vi "T2_Test_Frequency_Calibration_V2.vi"() -> ()   [LabVIEW 2020]
uses:
  <instrlib>/niFgen/niFgen.llb/niFgen Output Mode.ctl
  <instrlib>/niFgen/niFgen.llb/niFgen Waveform Type.ctl
  <instrlib>/niFgen/niFgen.llb/niFgen_ctl Trigger DigEdge - Edge Values (Ring).ctl
  <instrlib>/niFgen/niFgen.llb/niFgen_ctl Trigger Source Values (Ring).ctl
  <instrlib>/niFgen/niFgen.llb/niFgen Trigger Mode.ctl
  <instrlib>/niScope/Controls/niScope acquisition type.ctl
  <instrlib>/niScope/Controls/niScope trigger slope.ctl
  <instrlib>/niScope/Controls/niScope trigger source.ctl
  <vilib>/Utility/file.llb/Read Delimited Spreadsheet (DBL).vi
  <instrlib>/niFgen/niFgen.llb/niFgen Create Waveform (DBL).vi
  <instrlib>/niScope/Configure/Trigger/niScope Configure Trigger Edge.vi
  <instrlib>/niFgen/niFgen.llb/niFgen Configure Digital Edge Start Trigger.vi
  <instrlib>/niScope/Acquire/Fetch/niScope Fetch Cluster.vi
panel:
  out "Pulse Echos - Current Scan":waveform(dbl)(graph)={"t0"=timestamp(0 s since 1904-01-01), "dt"=0.0025142857142857146, "Y"=array[865 elements]} caption="Waveform Graph"
  out "Frequency List (MHz)":dbl[](array[numeric])
  out "Peaks":dbl[](array[numeric])
  in  "Pulse Train File":path=path "D:/Pulse Train - 4s Duration, 3170 Pulses, 1.25ms Tau.txt"
  in  "Starting Frequency":dbl=27440000.0 caption="Frequency" format="%.4p"
  out "Scan Number":i32=1
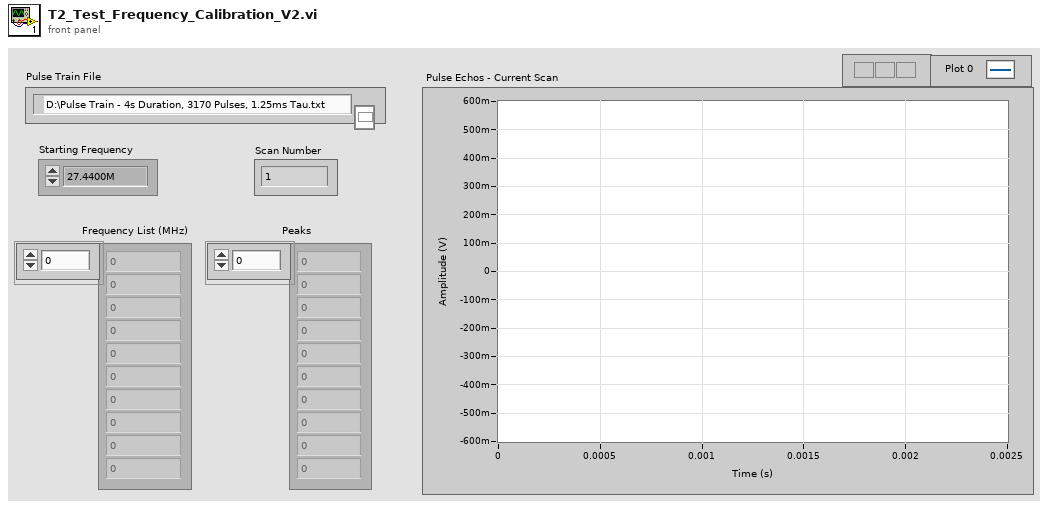
[diagram p1: front panel]
types:
  T1 = typedef "niFgen Output Mode.ctl" = u32
  T2 = typedef "niScope trigger source.ctl" = string
  T3 = typedef "niFgen_ctl Trigger Source Values (Ring).ctl" = string
  T4 = typedef "niScope trigger slope.ctl" = i32
  T5 = typedef "niScope acquisition type.ctl" = i32
  T6 = typedef "niFgen Trigger Mode.ctl" = i32
  T7 = typedef "niFgen_ctl Trigger DigEdge - Edge Values (Ring).ctl" = i32
  T8 = typedef "niFgen Waveform Type.ctl" = i32
  T9 = cluster{"relativeInitialX":dbl, "xIncrement":dbl, "wfm":dbl[]}
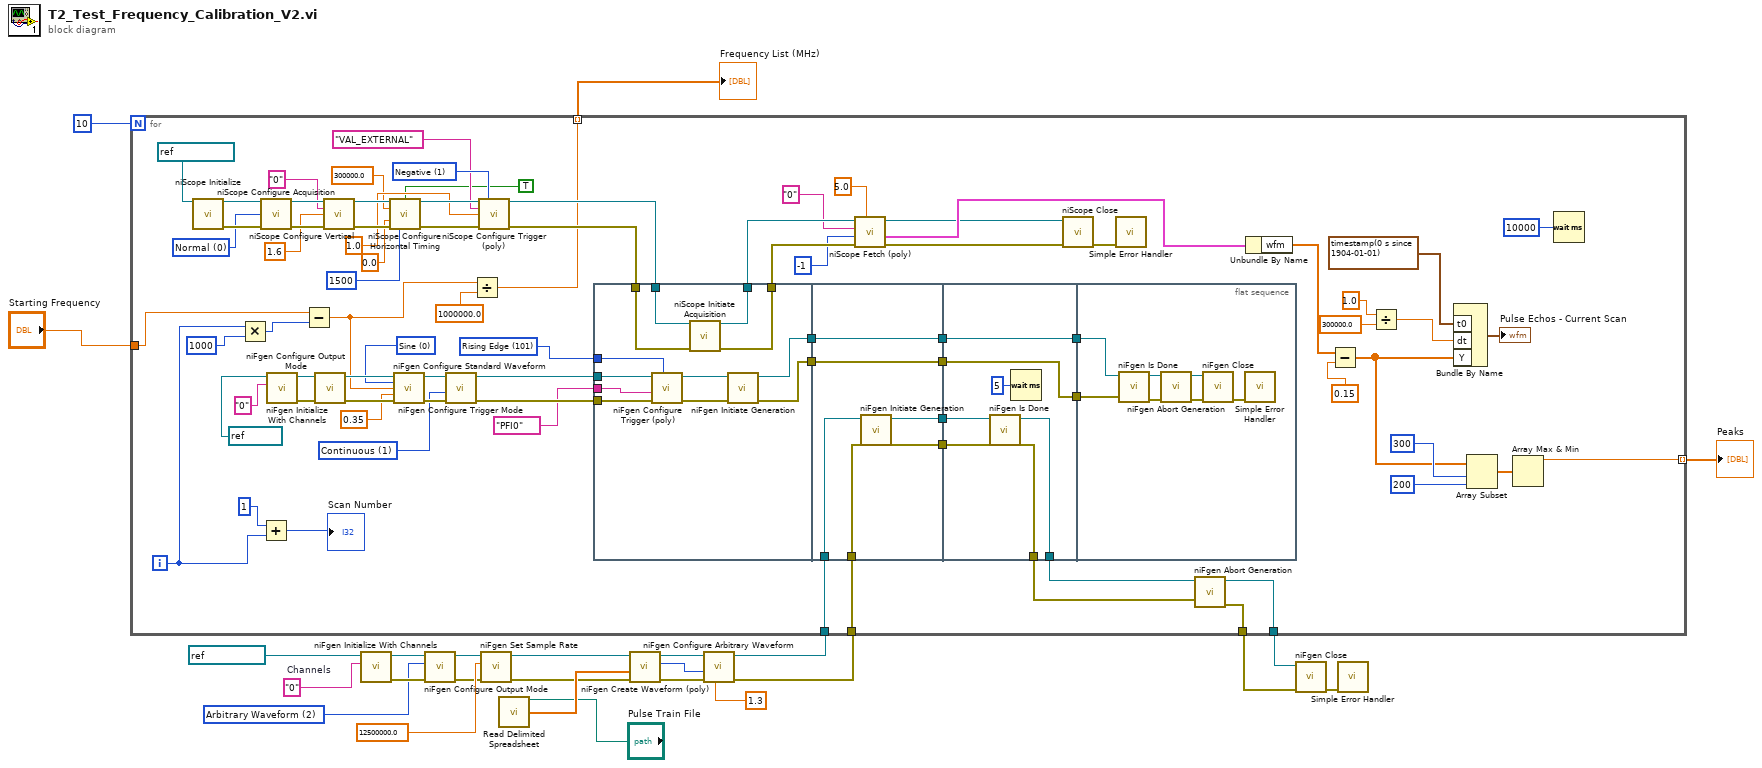
[diagram p0: block diagram]
diagram:
  w11 = "0"  # Channels
  w10 = T1 2 items=["Standard Function", "Frequency List", "Arbitrary Waveform", "Arbitrary Sequence", "Script"] ("output mode")
  n1 = call <instrlib>:"niFgen Initialize With Channels.vi"("Channel Name"=w11, "Resource Name"=refnum<k15> "PXI1Slot3" ("FGEN Resource Name 2")) -> ("error out"=w14:errorcluster, "Instrument Handle Out"=w15:refnum<k15>)  [unwired: 8 in]
  n2 = call <instrlib>:"niFgen Configure Output Mode.vi"("error in (no error)"=w14, "Output Mode (default: 0=Standard Function)"=w10, "Instrument Handle"=w15) -> ("error out"=w18:errorcluster, "Instrument Handle Out"=w17:refnum<k15>)  [unwired: 6 in]
  n3 = call <instrlib>:"niFgen Set Sample Rate.vi"("error in (no error)"=w18, "Sample Rate (Samp/s)"=12500000.0 ("Sample Rate"), "Instrument Handle"=w17) -> ("error out"=w21:errorcluster, "Instrument Handle Out"=w20:refnum<k15>)  [unwired: 7 in]
  n4 = call-poly <vilib>:"Read Delimited Spreadsheet.vi"("file path (dialog if empty)"="Pulse Train File") -> ("first row"=w22:dbl[])  [unwired: 9 in, 5 out]
  n5 = call-poly <instrlib>:"niFgen Create Waveform (poly).vi"("error in (no error)"=w21, "Waveform Data Array"=w22, "Instrument Handle"=w20) -> ("error out"=w24:errorcluster, "Waveform Handle"=w25:i32, "Instrument Handle Out"=w23:refnum<k15>)  [unwired: 6 in]
  n6 = call <instrlib>:"niFgen Configure Arbitrary Waveform.vi"("Gain"=1.3, "error in (no error)"=w24, "Waveform Handle"=w25, "Instrument Handle"=w23) -> ("error out"=w9:errorcluster, "Instrument Handle Out"=w8:refnum<k15>)  [unwired: 6 in]
  n7 = for {
    N: 10 ("Number of Scans") -> [_]
    tunnel: w9 -> [w90]
    tunnel: w8 -> [w89]
    tunnel: [w88] -> w6
    tunnel: [w87] -> w5
    tunnel: [w27] -> w3 mode=indexing
    tunnel: "Starting Frequency" -> [w45]
    tunnel: [w41] -> w1 mode=indexing
    i -> [w44]
    w75 = T4 1 items=["Positive", "Negative"] ("trigger slope")
    w76 = T5 0 items=["Normal"=0, "Flex Res"=1, "DDC"=3] ("acquisition Type")
    w93 = T6 1 items=["Single", "Continuous", "Stepped", "Burst"] ("Trigger Mode (default: 1=continuous)")
    w97 = T7 101 items=["Rising Edge"=101, "Falling Edge"=102] ("Edge (Rising)")
    w98 = T8 0 items=["Sine", "Square", "Triangle", "Ramp Up", "Ramp Down", "DC", "Noise", "User"] ("Waveform")
    n8 = call <instrlib>:"niScope Initialize.vi"("resource name"=refnum<k15> "PXI1Slot6") -> ("instrument handle"=w77:refnum<k15>, "error out"=w78:errorcluster)  [unwired: 13 in]
    n9 = Multiply(x=w44, y=1000) -> (x*y=w42:i32)
    n10 = call <instrlib>:"niScope Configure Acquisition.vi"("instrument handle"=w77, "acquisition Type"=w76, "error in"=w78) -> ("instrument handle out"=w80:refnum<k15>, "error out"=w81:errorcluster)  [unwired: 11 in]
    n11 = Add(x=1, y=w44) -> (x+y=→"Scan Number":i32)
    n12 = call <instrlib>:"niFgen Initialize With Channels.vi"("Channel Name"="0", "Resource Name"=refnum<k15> "Dev1" ("Sine Wave Module")) -> ("error out"=w103:errorcluster, "Instrument Handle Out"=w106:refnum<k15>)  [unwired: 8 in]
    n13 = Subtract(x=w45, y=w42) -> (x-y=w40:dbl)
    n14 = call <instrlib>:"niFgen Configure Output Mode.vi"("error in (no error)"=w103, "Instrument Handle"=w106) -> ("error out"=w102:errorcluster, "Instrument Handle Out"=w105:refnum<k15>)  [unwired: 7 in]
    n15 = call <instrlib>:"niScope Configure Vertical.vi"("instrument handle"=w80, "channels"="0", "vertical range"=1.6, "error in"=w81) -> ("instrument handle out"=w82:refnum<k15>, "error out"=w83:errorcluster)  [unwired: 10 in]
    n16 = call <instrlib>:"niScope Configure Horizontal Timing.vi"("instrument handle"=w82, "enforce realtime"=TRUE, "min sample rate"=300000.0, "reference position"=0.0, "error in"=w83, "min record length"=1500) -> ("instrument handle out"=w84:refnum<k15>, "error out"=w85:errorcluster)  [unwired: 8 in]
    n17 = call <instrlib>:"niFgen Configure Standard Waveform.vi"("Instrument Handle"=w105, "Waveform"=w98, "Frequency"=w40, "Amplitude"=0.35, "error in (no error)"=w102) -> ("Instrument Handle Out"=w104:refnum<k15>, "error out"=w101:errorcluster)  [unwired: 9 in]
    n18 = call <instrlib>:"niFgen Configure Trigger Mode.vi"("error in (no error)"=w101, "Trigger Mode (default: 1=continuous)"=w93, "Instrument Handle"=w104) -> ("error out"=w96:errorcluster, "Instrument Handle Out"=w94:refnum<k15>)  [unwired: 7 in]
    n19 = Divide(x=w40, y=1000000.0) -> (x/y=w41:dbl)
    n20 = call-poly <instrlib>:"niScope Configure Trigger (poly).vi"("instrument handle"=w84, "trigger slope"=w75, "trigger source"=T2 "VAL_EXTERNAL", "trigger level"=1.0, "error in"=w85) -> ("instrument handle out"=w69:refnum<k15>, "error out"=w68:errorcluster)  [unwired: 9 in]
    n21 = flat-sequence {
      tunnel: w97 -> [w117]
      tunnel: w96 -> [w116]
      tunnel: T3 "PFI0" ("Source") -> [w115]
      tunnel: w94 -> [w114]
      tunnel: w69 -> [w112]
      tunnel: w68 -> [w111]
      tunnel: [w110] -> w67
      tunnel: [w109] -> w66
      tunnel: [w108] -> w56
      tunnel: [w107] -> w53
      tunnel: w90 -> [w124]
      tunnel: w89 -> [w123]
      tunnel: [w122] -> w60
      tunnel: [w121] -> w59
      tunnel: [w120] -> w57
      tunnel: w56 -> [w120]
      tunnel: [w119] -> w54
      tunnel: w53 -> [w119]
      tunnel: [w130] -> w92
      tunnel: [w129] -> w91
      tunnel: w60 -> [w128]
      tunnel: w59 -> [w127]
      tunnel: [w126] -> w58
      tunnel: w57 -> [w126]
      tunnel: [w125] -> w55
      tunnel: w54 -> [w125]
      tunnel: w58 -> [w133]
      tunnel: w55 -> [w132]
      frame #0 {
        n22 = call-poly <instrlib>:"niFgen Configure Trigger (poly).vi"("Edge (Rising)"=w117, "error in (no error)"=w116, "Source"=w115, "Instrument Handle"=w114) -> ("error out"=w113:errorcluster, "Instrument Handle Out"=w118:refnum<k15>)  [unwired: 6 in]
        n23 = call <instrlib>:"niScope Initiate Acquisition.vi"("instrument handle"=w112, "error in"=w111) -> ("instrument handle out"=w110:refnum<k15>, "error out"=w109:errorcluster)  [unwired: 12 in]
        n24 = call <instrlib>:"niFgen Initiate Generation.vi"("error in (no error)"=w113, "Instrument Handle"=w118) -> ("error out"=w107:errorcluster, "Instrument Handle Out"=w108:refnum<k15>)  [unwired: 8 in]
      }
      frame #1 {
        n25 = call <instrlib>:"niFgen Initiate Generation.vi"("error in (no error)"=w124, "Instrument Handle"=w123) -> ("error out"=w121:errorcluster, "Instrument Handle Out"=w122:refnum<k15>)  [unwired: 8 in]
      }
      frame #2 {
        n26 = call <instrlib>:"niFgen Is Done.vi"("error in (no error)"=w127, "Instrument Handle"=w128) -> ("error out"=w130:errorcluster, "Instrument Handle Out"=w129:refnum<k15>)  [unwired: 7 in, 1 out]
        n27 = Wait (ms)(milliseconds to wait=u32 5) -> ()  [unwired: 1 out]
      }
      frame #3 {
        n28 = call <instrlib>:"niFgen Is Done.vi"("error in (no error)"=w132, "Instrument Handle"=w133) -> ("error out"=w136:errorcluster, "Instrument Handle Out"=w135:refnum<k15>)  [unwired: 7 in, 1 out]
        n29 = call <instrlib>:"niFgen Abort Generation.vi"("error in (no error)"=w136, "Instrument Handle"=w135) -> ("error out"=w137:errorcluster, "Instrument Handle Out"=w138:refnum<k15>)  [unwired: 8 in]
        n30 = call <instrlib>:"niFgen Close.vi"("error in (no error)"=w137, "Instrument Handle"=w138) -> ("error out"=w134:errorcluster)  [unwired: 9 in]
        n31 = call <vilib>:"Simple Error Handler.vi"("error in (no error)"=w134) -> ()  [unwired: 4 in, 5 out]
      }
    }
    n32 = call-poly <instrlib>:"niScope Fetch (poly).vi"("timeout"=5.0, "error in"=w66, "numSamples"=-1, "channels"="0", "instrument handle"=w67) -> ("error out"=w47:errorcluster, "waveform"=w50:T9, "instrument handle out"=w48:refnum<k15>)  [unwired: 3 in, 1 out]
    n33 = call <instrlib>:"niScope Close.vi"("instrument handle"=w48, "error in"=w47) -> ("error out"=w86:errorcluster)  [unwired: 13 in]
    n34 = call <vilib>:"Simple Error Handler.vi"("error in (no error)"=w86) -> ()  [unwired: 4 in, 5 out]
    n35 = call <instrlib>:"niFgen Abort Generation.vi"("error in (no error)"=w92, "Instrument Handle"=w91) -> ("error out"=w88:errorcluster, "Instrument Handle Out"=w87:refnum<k15>)  [unwired: 8 in]
    n36 = Unbundle By Name(w50) -> ("wfm"=w29:dbl[])
    n37 = Subtract(x=w29, y=0.15) -> (x-y=w26:dbl[])
    n38 = Divide(x=1.0, y=300000.0) -> (x/y=w33:dbl)
    n39 = Bundle By Name("t0"=timestamp(0 s since 1904-01-01), "dt"=w33, "Y"=w26) -> (→"Pulse Echos - Current Scan":waveform(dbl))  [unwired: 1 in]
    n40 = Array Subset(array=w26, index=300 ("y"), length=200 ("y")) -> (w31:dbl[])
    n41 = Array Max & Min(array=w31) -> (max value=w27:dbl)  [unwired: 3 out]
    n42 = Wait (ms)(milliseconds to wait=u32 10000) -> ()  [unwired: 1 out]
  }
  "Peaks" <- w3
  "Frequency List (MHz)" <- w1
  n43 = call <instrlib>:"niFgen Close.vi"("error in (no error)"=w6, "Instrument Handle"=w5) -> ("error out"=w7:errorcluster)  [unwired: 9 in]
  n44 = call <vilib>:"Simple Error Handler.vi"("error in (no error)"=w7) -> ()  [unwired: 4 in, 5 out]
